vi "Set ID.vi"(8 "error in (no error)":errorcluster, 10 "ID":i32, 11 "Connection in":refnum<class "Connection.lvclass">) -> (0 "error out":errorcluster, 3 "Connection out":refnum<class "Connection.lvclass">)   [LabVIEW 2020, in "Parallel Block.lvlib" / "Connection.lvclass"]
uses:
  Connection.lvclass
  Connection.lvclass/Connection.ctl
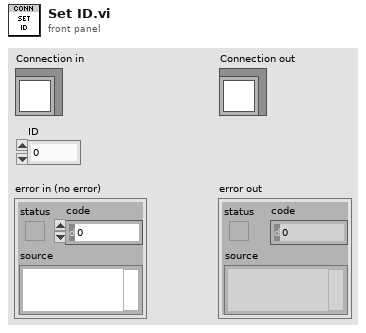
[diagram p1: front panel]
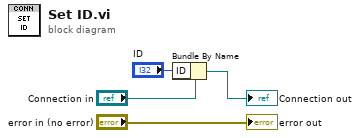
[diagram p0: block diagram]
diagram:
  n1 = Bundle By Name(cluster="Connection in", "ID"="ID") -> (→"Connection out":refnum<class "Connection.lvclass">)
  "error out" <- "error in (no error)"
